vi "CSC_Config1.vi"(8 "error in (no error)":errorcluster, 11 "C-Alex in":refnum<class "CableSerialChain.lvclass">) -> (0 "error out":errorcluster, 3 "C-Alex out":refnum<class "CableSerialChain.lvclass">)   [LabVIEW 2014]
uses:
  CableSerialChain.lvclass
  Body/PointOnBody.ctl
  Body/Bodies.lvclass
panel:
  in  "Shank":T2={"Center of Mass in Cuff Coord Sys"={"Coord4"=[-9e-06, -0.001261, 0.085739, 1.0], "ID"=4}, "Mass"=0.717532, "Cable Attachment Points in Cuff Coord Sys"=[{"Coord4"=[-0.036195, 0.12365173, 0.01784759, 1.0], "ID"=6}, {"Coord4"=[0.036195, -0.12365173, 0.01784759, 1.0], "ID"=7}]} {"Mass" format="%#_13g"}
  in  "Thigh":T2={"Center of Mass in Cuff Coord Sys"={"Coord4"=[-0.001154, 9e-06, 0.110262, 1.0], "ID"=3}, "Mass"=0.783684, "Cable Attachment Points in Cuff Coord Sys"=[{"Coord4"=[0.16243322, -0.036195, 0.01632515, 1.0], "ID"=5}, {"Coord4"=[0.16167122, -0.036195, 0.02390696, 1.0], "ID"=6}, {"Coord4"=[-0.16167122, 0.036195, 0.02390696, 1.0], "ID"=7}, {"Coord4"=[-0.16243322, 0.036195, 0.01632515, 1.0], "ID"=8}]} {"Mass" format="%#_13g"}
  in  "Pelvis":T3={"Center of Mass in Cuff Coord Sys"={"Coord4"=[0.0, 0.0, 0.0, 1.0], "ID"=0}, "Mass"=0.0, "Cable Attachment Cuff Coord Sys"=[{"Coord4"=[0.276524, 0.0, 0.007338, 1.0], "ID"=5}, {"Coord4"=[0.276112, 0.0, 0.014947, 1.0], "ID"=6}, {"Coord4"=[-0.276112, 0.0, 0.014947, 1.0], "ID"=7}, {"Coord4"=[-0.276524, 0.0, 0.007338, 1.0], "ID"=8}]} {"Mass" format="%#_13g"}
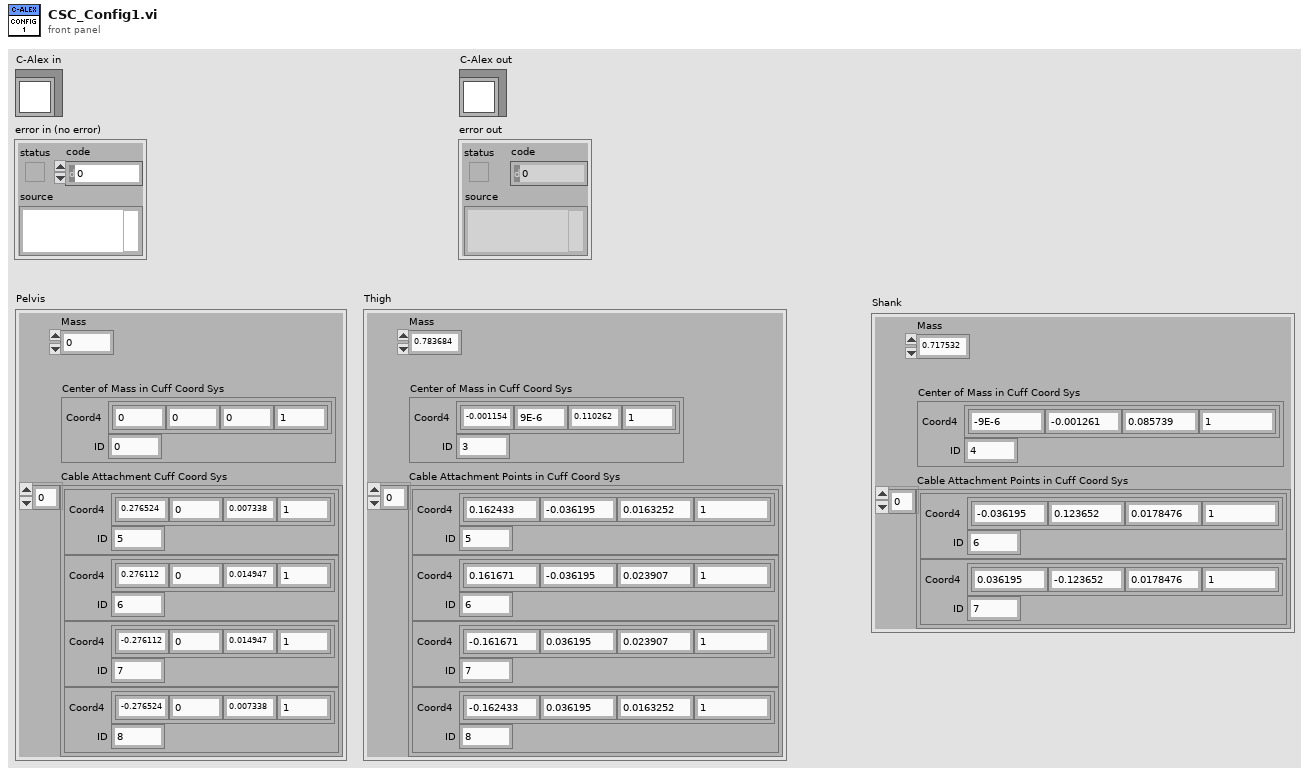
[diagram p1: front panel]
types:
  T1 = typedef "Bodies.lvclass/PointOnBody.ctl" = cluster{"Coord4":dbl[], "ID":i32}
  T2 = cluster{"Center of Mass in Cuff Coord Sys":T1, "Mass":dbl, "Cable Attachment Points in Cuff Coord Sys":T1[]}
  T3 = cluster{"Center of Mass in Cuff Coord Sys":T1, "Mass":dbl, "Cable Attachment Cuff Coord Sys":T1[]}
  T4 = cluster{"PelvicCuffOffset(m)":dbl, "ThighCuffOffset(m)":dbl, "ShankCuffOffset(m)":dbl}
  T5 = cluster{"Thigh Length (m)":dbl, "Shank Length (m)":dbl}
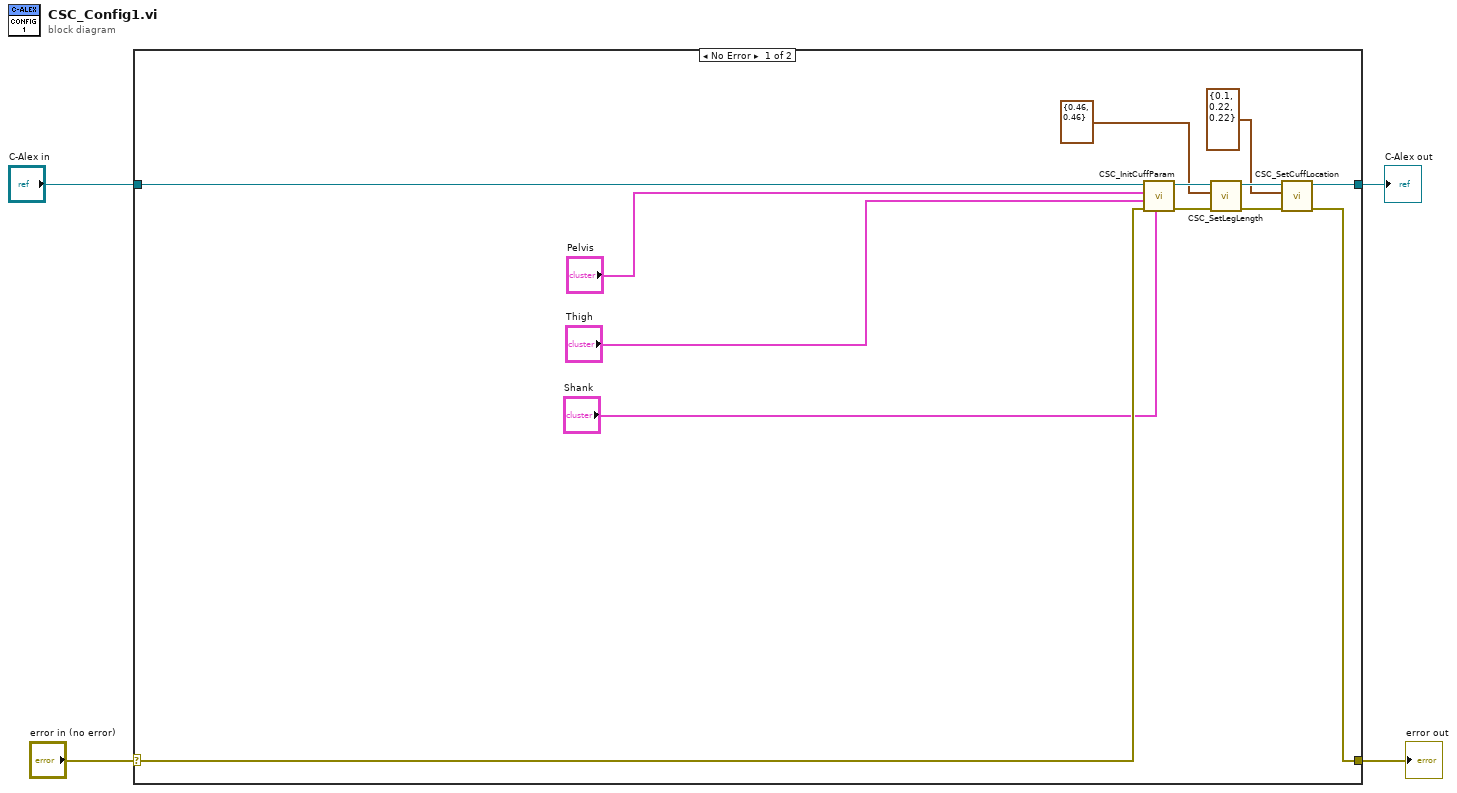
[diagram p0: block diagram]
diagram:
  n1 = case shown="No Error" "error in (no error)" {
    selector: "error in (no error)" -> [w16 w19]
    tunnel: [w7 w19] -> w3
    tunnel: [w8 w18] -> w1
    tunnel: "C-Alex in" -> [w17 w18]
    frame No Error {
      n2 = call "CSC_InitCuffParam.vi"("Shank"="Shank", "error in (no error)"=w16, "Thigh"="Thigh", "Pelvis"="Pelvis", "C-Alex in"=w17) -> ("error out"=w12:errorcluster, "C-Alex out"=w11:refnum<class "CableSerialChain.lvclass">)  [unwired: 5 in]
      n3 = call "CSC_SetLegLength.vi"("error in (no error)"=w12, "LegLength"=T5 {"Thigh Length (m)"=0.46, "Shank Length (m)"=0.46}, "C-Alex in"=w11) -> ("error out"=w10:errorcluster, "C-Alex out"=w9:refnum<class "CableSerialChain.lvclass">)  [unwired: 7 in]
      n4 = call "CSC_SetCuffLocation.vi"("error in (no error)"=w10, "Cuff Location"=T4 {"PelvicCuffOffset(m)"=0.1, "ThighCuffOffset(m)"=0.22, "ShankCuffOffset(m)"=0.22}, "C-Alex in"=w9) -> ("error out"=w7:errorcluster, "C-Alex out"=w8:refnum<class "CableSerialChain.lvclass">)  [unwired: 7 in]
    }
    frame Error {
    }
  }
  "error out" <- w3
  "C-Alex out" <- w1
